vi "cvt_Enum_TagList.vi"(8 "error in (no error)":errorcluster, 9 "Tag Name":string, 10 "Tag List":T1[](array[typedef]), 11 "Method":T3=enum."getindex") -> (0 "error out":errorcluster, 1 "Index":i32, 2 "Default Data":i32[](array[numeric]), 3 "Tag Description":string, 4 "Enum Values":string[](array[string]), 5 "Enum Tag List":T1[](array[typedef]))   [LabVIEW 2020, in "Current Value Table(Rebuild).lvlib"]
uses:
  Current Value Table(Rebuild).lvlib
  TypeDefs/cvt_TagList Methods.ctl
  TypeDefs/cvt_Tag Configuration.ctl
  TypeDefs/cvt_Data Types.ctl
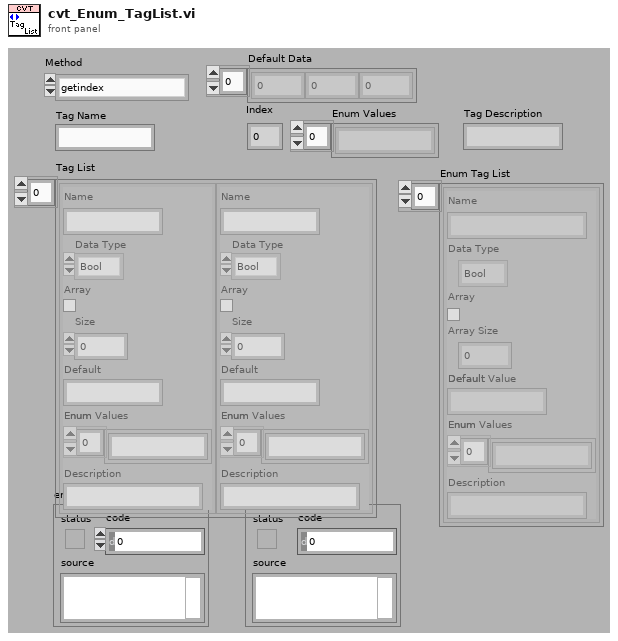
[diagram p1: front panel]
types:
  T1 = typedef "Current Value Table(Rebuild).lvlib/cvt_Tag Configuration.ctl" = cluster{"Name":string, "Data Type":T2, "Array":bool, "Size":u32, "Default":string, "Enum":string[], "Description":string}
  T2 = typedef "Current Value Table(Rebuild).lvlib/cvt_Data Types.ctl" = enum16{"Bool", "U8", "I32", "Double", "String", "Enum"}
  T3 = typedef "Current Value Table(Rebuild).lvlib/cvt_TagList Methods.ctl" = enum16{"init", "getindex", "getdesc", "getlist"}
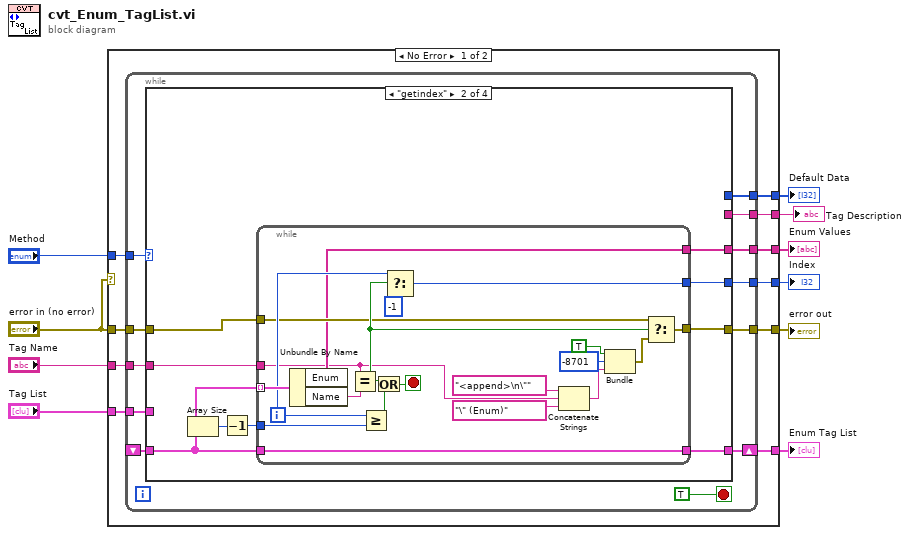
[diagram p0: block diagram]
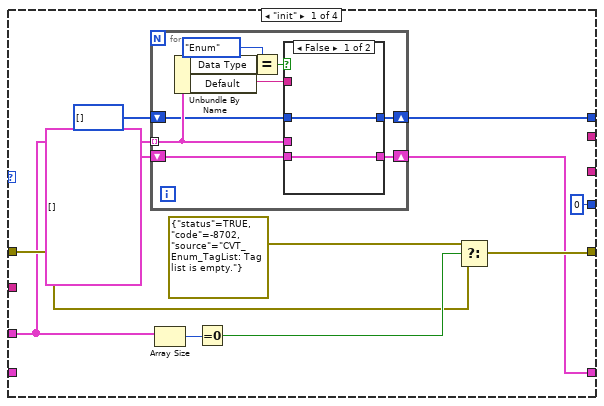
[diagram p2: hidden frame]
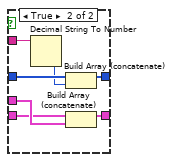
[diagram p3: hidden frame]
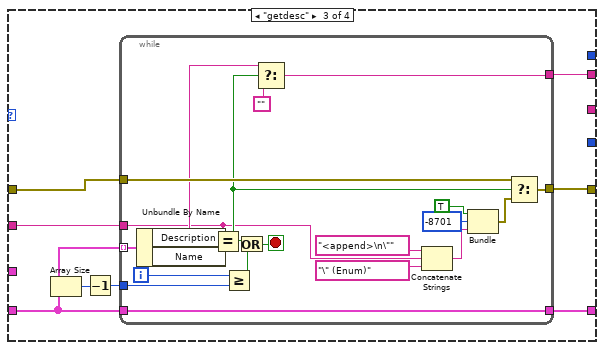
[diagram p4: hidden frame]
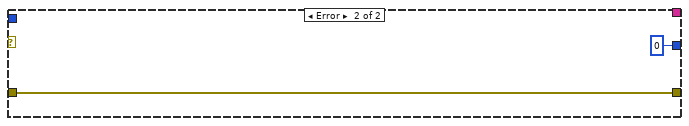
[diagram p6: hidden frame]
diagram:
  n1 = case shown="No Error" "error in (no error)" {
    tunnel: "Method" -> [w20 _]
    tunnel: "Tag Name" -> [w19 _]
    tunnel: [w18 w122] -> w8
    tunnel: "error in (no error)" -> [w17 w122]
    tunnel: "Tag List" -> [w16 _]
    tunnel: [w15 0 ("f")] -> w5
    tunnel: [w14 _] -> w4
    tunnel: [w13 _] -> w3
    tunnel: [w12 _] -> w2
    tunnel: [w11 _] -> w1
    frame No Error {
      n2 = while {
        tunnel: w20 -> [w31]
        tunnel: w19 -> [w30]
        tunnel: w17 -> [w29]
        tunnel: [w28] -> w18
        tunnel: w16 -> [w25]
        shift-right: [w27] -> w11
        shift-left: _ -> [w26]
        tunnel: [w24] -> w15
        tunnel: [w23] -> w14
        tunnel: [w22] -> w13
        tunnel: [w21] -> w12
        stop <- TRUE stop-if-true
        n3 = case shown="\"getindex\"" w31 {
          tunnel: w30 -> [_ w70 w98 _]
          tunnel: w29 -> [w40 w64 w92 w119]
          tunnel: [w42 w65 w93 w119] -> w28
          tunnel: [w36 w67 w95 w120] -> w27
          tunnel: w26 -> [_ w66 w94 w120]
          tunnel: w25 -> [w37 _ _ _]
          tunnel: [0 ("f") w63 _ _] -> w24
          tunnel: [w34 _ _ _] -> w23
          tunnel: [_ w62 _ _] -> w22
          tunnel: [_ _ w91 _] -> w21
          frame "init" {
            n4 = for {
              tunnel: w37 -> [w48] mode=indexing
              shift-right: [w46] -> w36
              shift-left: T1[] [] -> [w47]
              shift-right: [w44] -> w34
              shift-left: i32[] [] -> [w45]
              n5 = Unbundle By Name(w48) -> ("Data Type"=w52:T2, "Default"=w49:string)
              n6 = Equal?(x=cvt_Data_Types."Enum", y=w52) -> (x = y?=w51:bool)
              n7 = case shown="False" w51 {
                tunnel: w49 -> [_ w56]
                tunnel: w45 -> [w53 w61]
                tunnel: [w53 w60] -> w44
                tunnel: w48 -> [_ w59]
                tunnel: w47 -> [w54 w58]
                tunnel: [w54 w57] -> w46
                frame False {
                }
                frame True {
                  n8 = Decimal String To Number(string=w56) -> (number=w55:i32)  [unwired: 3 out]
                  n9 = Build Array (concatenate)(w61, w55) -> (w60:i32[])
                  n10 = Build Array (concatenate)(w58, w59) -> (w57:T1[])
                }
              }
            }
            n11 = Array Size(array=w37) -> (size(s)=w43:i32)
            n12 = Equal To 0?(x=w43) -> (x = 0?=w41:bool)
            n13 = Select(t=errorcluster {"status"=TRUE, "code"=-8702, "source"="CVT_Enum_TagList: Tag list is empty."} ("f"), s=w41, f=w40) -> (s? t:f=w42:errorcluster)
          }
          frame "getindex" {
            n14 = Array Size(array=w66) -> (size(s)=w69:i32)
            n15 = Decrement(x=w69) -> (x-1=w68:i32)
            n16 = while {
              tunnel: w66 -> [w90] mode=indexing
              tunnel: w70 -> [w71]
              tunnel: w68 -> [w88]
              tunnel: [w79] -> w63
              tunnel: [w82] -> w67
              tunnel: w66 -> [w82]
              tunnel: [w81] -> w65
              tunnel: w64 -> [w80]
              tunnel: [w78] -> w62
              i -> [w85]
              stop <- w86 stop-if-true
              n17 = Unbundle By Name(w90) -> ("Enum"=w78:string[], "Name"=w89:string)
              n18 = Equal?(x=w71, y=w89) -> (x = y?=w83:bool)
              n19 = Greater Or Equal?(x=w85, y=w88) -> (x >= y?=w87:bool)
              n20 = Or(x=w83, y=w87) -> (x .or. y?=w86:bool)
              n21 = Select(t=w85, s=w83, f=-1) -> (s? t:f=w79:i32)
              n22 = Concatenate Strings("<append>\n\"" ("source"), w71, "\" (Enum)" ("source")) -> (w74:string)
              n23 = Bundle("status"=TRUE, "code"=-8701, w74) -> (w72:cluster{"status":bool, "code":i32, string})  [unwired: 1 out]
              n24 = Select(t=w80, s=w83, f=w72) -> (s? t:f=w81:errorcluster)
            }
          }
          frame "getdesc" {
            n25 = Array Size(array=w94) -> (size(s)=w97:i32)
            n26 = Decrement(x=w97) -> (x-1=w96:i32)
            n27 = while {
              tunnel: w94 -> [w118] mode=indexing
              tunnel: w98 -> [w99]
              tunnel: w96 -> [w116]
              tunnel: [w112] -> w95
              tunnel: w94 -> [w112]
              tunnel: [w111] -> w93
              tunnel: w92 -> [w110]
              tunnel: [w107] -> w91
              i -> [w113]
              stop <- w114 stop-if-true
              n28 = Unbundle By Name(w118) -> ("Description"=w108:string, "Name"=w117:string)
              n29 = Equal?(x=w99, y=w117) -> (x = y?=w109:bool)
              n30 = Greater Or Equal?(x=w113, y=w116) -> (x >= y?=w115:bool)
              n31 = Or(x=w109, y=w115) -> (x .or. y?=w114:bool)
              n32 = Select(t=w108, s=w109, f="") -> (s? t:f=w107:string)
              n33 = Concatenate Strings("<append>\n\"" ("source"), w99, "\" (Enum)" ("source")) -> (w104:string)
              n34 = Bundle("status"=TRUE, "code"=-8701, w104) -> (w100:cluster{"status":bool, "code":i32, string})  [unwired: 1 out]
              n35 = Select(t=w110, s=w109, f=w100) -> (s? t:f=w111:errorcluster)
            }
          }
          frame "getlist" {
          }
        }
      }
    }
    frame Error {
    }
  }
  "error out" <- w8
  "Index" <- w5
  "Default Data" <- w4
  "Enum Values" <- w3
  "Tag Description" <- w2
  "Enum Tag List" <- w1
